vi "test Action Update Set Point-SetPoint10.vi"() -> ()   [LabVIEW 2018, in "Action Update Set Point.lvclass"]
uses:
  Action Update Set Point.lvclass
  E:/Program Files (x86)/National Instruments/Circuit Design Suite 14.1/LabVIEW 2018/vi.lib/addons/_JKI Toolkits/VI Tester/TestCase.llb/TestCase.lvclass
  <vilib>/addons/_JKI Toolkits/VI Tester/TestCase.llb/TestCase.lvclass
  Libraries/Thermal Chamber Controller_DQMH/Thermal Chamber Controller_DQMH.lvlib
  Libraries/Thermal Chamber Response Simulator/Thermal Chamber Response Simulator.lvlib
panel:
  out "TestCase out":refnum<class "TestCase.lvclass">
  in  "TestCase in":refnum<class "Action Update Set Point.lvclass">
  out "error out":errorcluster
  in  "error in (no error)":errorcluster
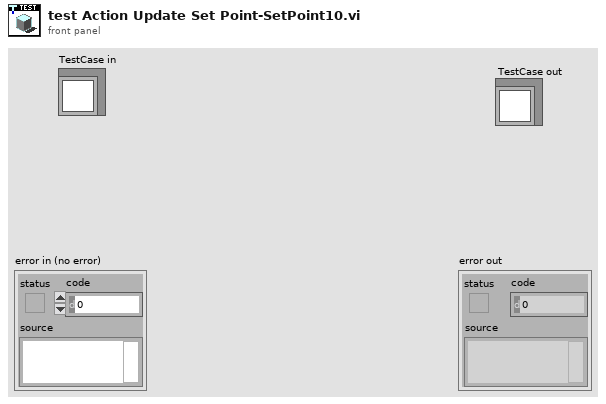
[diagram p1: front panel]
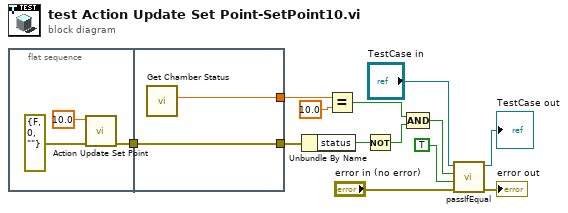
[diagram p0: block diagram]
diagram:
  n1 = flat-sequence {
    tunnel: [w16] -> w13
    tunnel: [w18] -> w2
    tunnel: w13 -> [w18]
    tunnel: [w17] -> w1
    frame #0 {
      n2 = call "Action Update Set Point.vi"("error in (no error)"=errorcluster {"status"=FALSE, "code"=0, "source"=""}, "Temperature Set Point"=10.0) -> ("error out"=w16:errorcluster)  [unwired: 9 in]
    }
    frame #1 {
      n3 = call "Get Chamber Status.vi"() -> ("Temperature Set Point (deg C)"=w17:dbl)  [unwired: 6 in, 5 out]
    }
  }
  n4 = Unbundle By Name(w2) -> ("status"=w5:bool)
  n5 = Equal?(x=w1, y=10.0) -> (x = y?=w6:bool)
  n6 = Not(x=w5) -> (.not. x?=w4:bool)
  n7 = Compound Arithmetic op=AND(w6, w4) -> (w3:bool)
  n8 = call-dynamic "passIfEqual.vi"("error in (no error)"="error in (no error)", "y"=TRUE, "x"=w3, "TestCase in"="TestCase in") -> ("error out"=→"error out":errorcluster, "TestCase out"=→"TestCase out":refnum<class "Action Update Set Point.lvclass">)  [unwired: 6 in]
